vi "MathCad_File_Close.vi"(8 "error in (no error)":errorcluster, 11 "Mathcad Worksheet":refnum<k7>) -> (0 "error out":errorcluster)   [LabVIEW 2015]
doc: "Closes a Mathcad file reference that was opened by Mathcad_File_Open.vi\n\nInputs\nWorksheet Reference- Reference to the opened Mathcad Worksheet Class outputted by the Mathcad_File_Open.vi\n\nError In -Error Cluster\n\nOutputs\nError Out- Error Cluster"
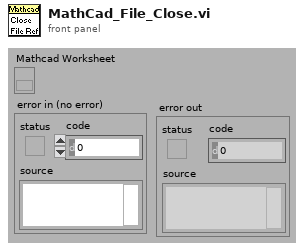
[diagram p1: front panel]
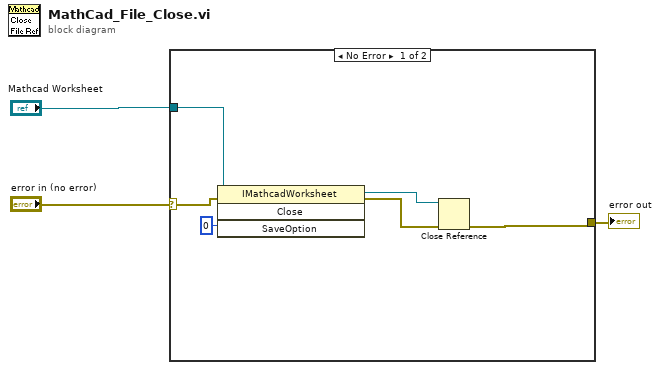
[diagram p0: block diagram]
diagram:
  n1 = case shown="No Error" "error in (no error)" {
    selector: "error in (no error)" -> [w4 w10]
    tunnel: [w7 w10] -> w3
    tunnel: "Mathcad Worksheet" -> [w5 _]
    frame No Error {
      n2 = invoke class="IMathcadWorksheet" method="Close"(reference=w5, error in=w4, "SaveOption"=0) -> (reference out=w6:refnum<k7>, error out=w8:errorcluster)  [unwired: 1 in, 2 out]
      n3 = Close Reference(reference=w6, error in (no error)=w8) -> (error out=w7:errorcluster)
    }
    frame Error {
    }
  }
  "error out" <- w3
